vi "initTempConfig.vi"() -> ()   [LabVIEW 2012]
uses:
  <vilib>/Utility/error.llb/DialogType.ctl
panel:
  out "stripped path":path
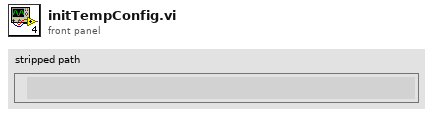
[diagram p1: front panel]
types:
  T1 = typedef "DialogType.ctl" = u16
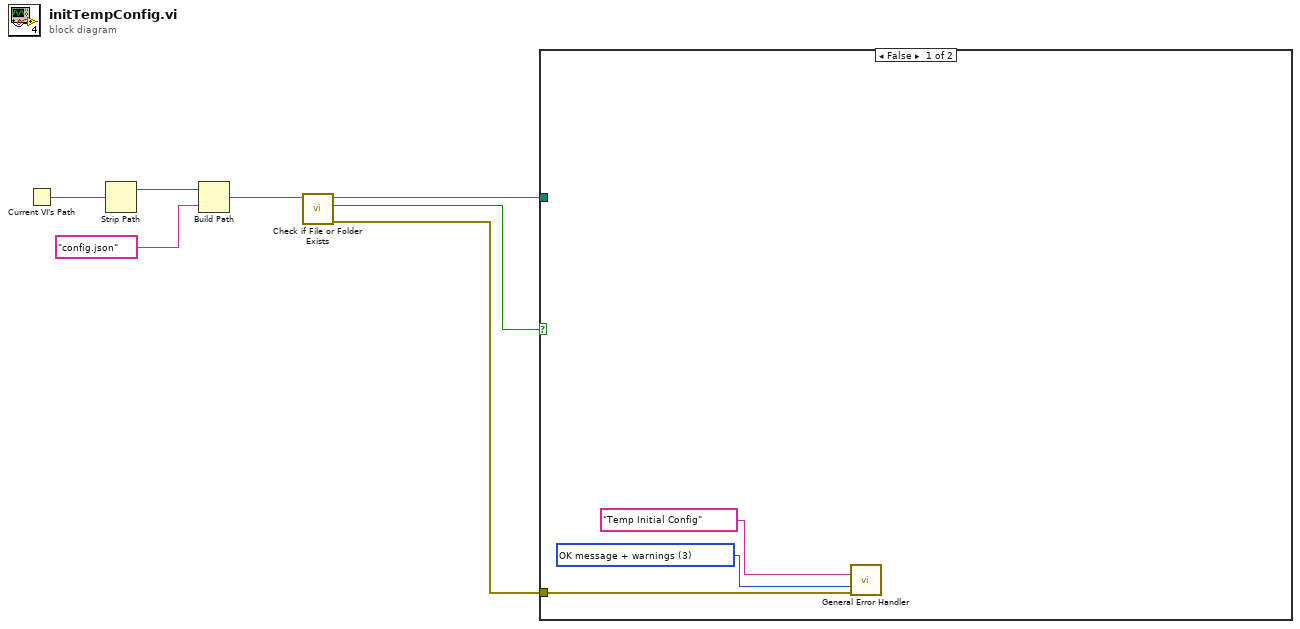
[diagram p0: block diagram]
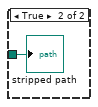
[diagram p2: hidden frame]
diagram:
  n1 = Current VI's Path() -> (path=w7:path)
  n2 = Strip Path(path=w7) -> (stripped path=w6:path)  [unwired: 1 out]
  n3 = Build Path(base path=w6, name or relative path="config.json") -> (appended path=w4:path)
  n4 = call <vilib>:"Check if File or Folder Exists.vi"("path"=w4) -> ("error out"=w1:errorcluster, "file or folder exists?"=w2:bool, "dup path"=w3:path)  [unwired: 8 in]
  n5 = case shown="False" w2 {
    tunnel: w3 -> [_ w11]
    tunnel: w1 -> [w10 _]
    frame False {
      w9 = T1 3 items=["no dialog", "OK message", "continue or stop message", "OK message + warnings", "continue/stop + warnings"] ("type of dialog (OK msg:1)")
      n6 = call <vilib>:"General Error Handler.vi"("[error source] (\" \")"="Temp Initial Config" ("[error source] (\" \")"), "type of dialog (OK msg:1)"=w9, "error in (no error)"=w10) -> ()  [unwired: 8 in, 5 out]
    }
    frame True {
      "stripped path" <- w11
    }
  }
